vi "FPGA_Main_R3.vi"() -> ()   [LabVIEW 2018]
uses:
  Data Def/FPGA_I2C Loop State.ctl
  <vilib>/rvi/Emulation/niFpgaGetClockAttributes.vi
  <vilib>/rvi/Emulation/niFpgaSctlEmulationGetInTimedLoop.vi
  <vilib>/rvi/Emulation/niFpgaEmulationReportErrorSimple.vi
  <vilib>/IEDriver/SPIandI2C/FPGA/Private/Initialize Port (I2C).vi
  <vilib>/IEDriver/SPIandI2C/FPGA/Private/Configure Port (I2C).vi
  <vilib>/IEDriver/SPIandI2C/FPGA/Private/Read Port (I2C).vi
  <vilib>/IEDriver/SPIandI2C/FPGA/Private/Arm Port (I2C).vi
  <vilib>/IEDriver/SPIandI2C/FPGA/Private/Write Port (I2C).vi
  <vilib>/rvi/Emulation/niFpgaProcessEmulError.vi
  <vilib>/rvi/interface/RandomDataEmulation/niFpgaRandomDataHandleErrors.vi
  <vilib>/rvi/Emulation/niFpgaCriticalErrorInLSC.vi
  <vilib>/IEDriver/SPIandI2C/FPGA/Private/IP Port (I2C).vi
  <vilib>/rvi/DataTransferAndStorage/Container/XNode/niFpgaContainer.xnode
  <vilib>/rvi/interface/RandomDataEmulation/nirviRandomDataFpgaReadWriteTemplate.vi
  <vilib>/IEDriver/SPIandI2C/FPGA/Library/IP SPI&I2C.lvlib
panel:
  out "Count":u32
  out "I2C Loop State View":T1
  out "Over":bool
  in  "Auto Read Count":u32
  out "Overflow":bool
  in  "I2C Loop State":T1
  out "Done":bool
  in  "Command Data":T2 {"Command (Write & Read)" items=["Write & Read", "Write", "Read"]}
  out "Actual Rate (Hz)":u32
  in  "I2C Protocol Input Data":u8
  out "I2C Protocol Output Data":u8
  in  "I2C Protocol Configure":T3
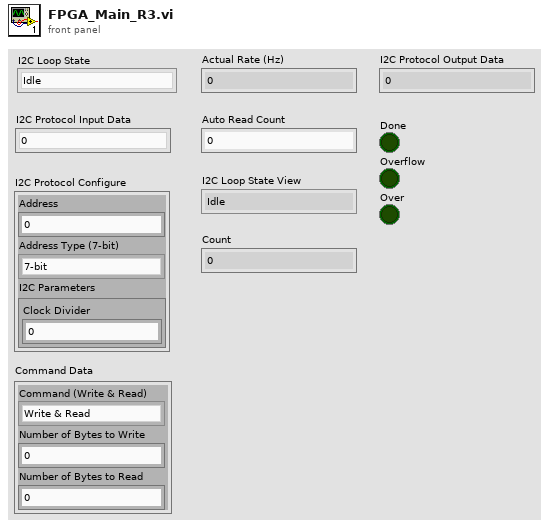
[diagram p1: front panel]
types:
  T1 = typedef "FPGA_I2C Loop State.ctl" = enum16{"Idle", "Set Idle", "Config", "Read", "Write", "Arm", "Auto Run", "Auto Config", "Auto Write", "Auto Arm", "Auto Read", "Auto Check"}
  T2 = cluster{"Command (Write & Read)":u8, "Number of Bytes to Write":u16, "Number of Bytes to Read":u16}
  T3 = cluster{"Address":u16, "Address Type (7-bit)":enum16{"7-bit", "10-bit"}, "I2C Parameters":cluster{"Clock Divider":u32}}
  T4 = typedef "IP SPI&I2C.lvlib/Private Data (I2C).ctl" = cluster{"Arm Trigger":refnum<k21>, "API to IP Data":refnum<k21>, "IP to API Data":refnum<k21>, "Configuration Register":refnum<k21>, "Configuration Lock":refnum<k21>}
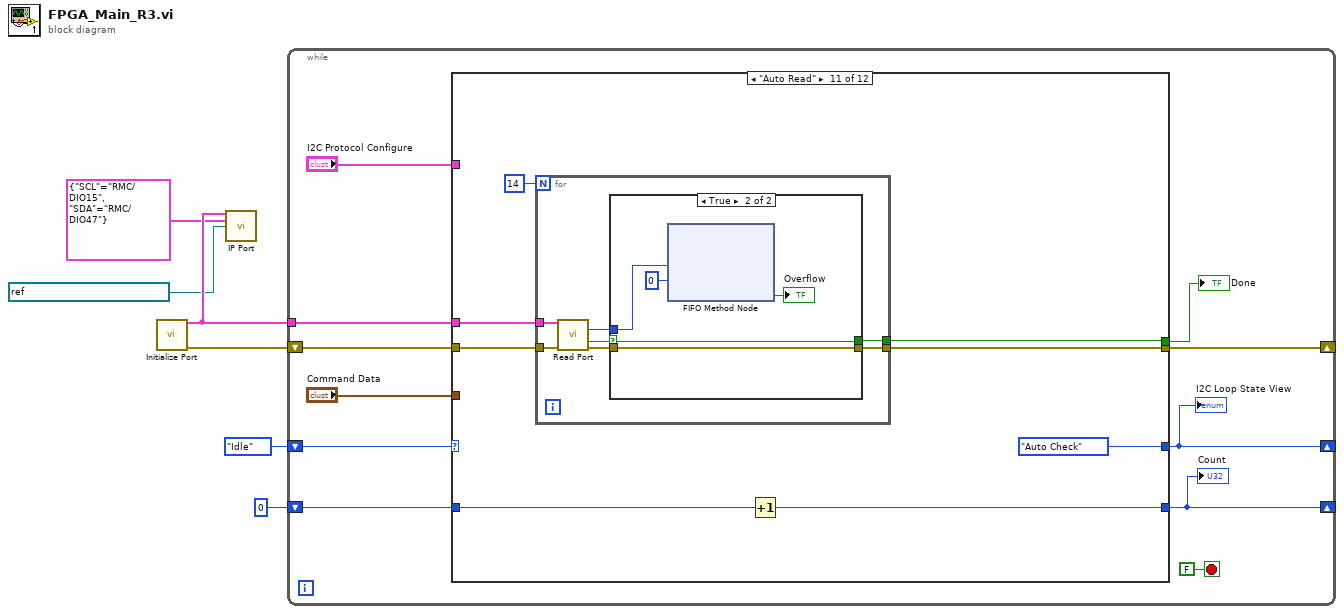
[diagram p0: block diagram]
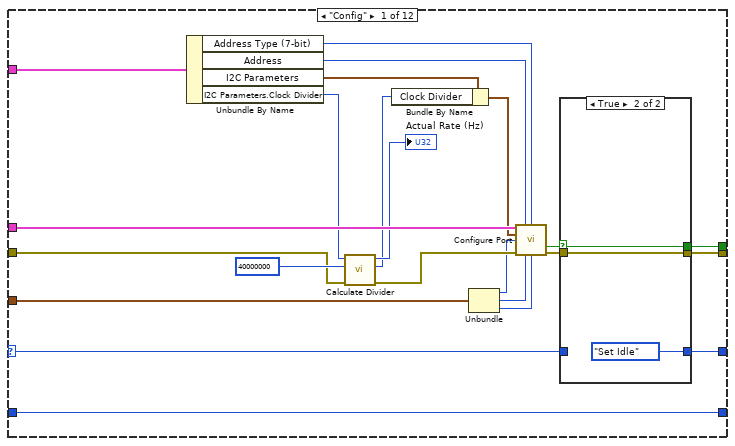
[diagram p2: hidden frame]
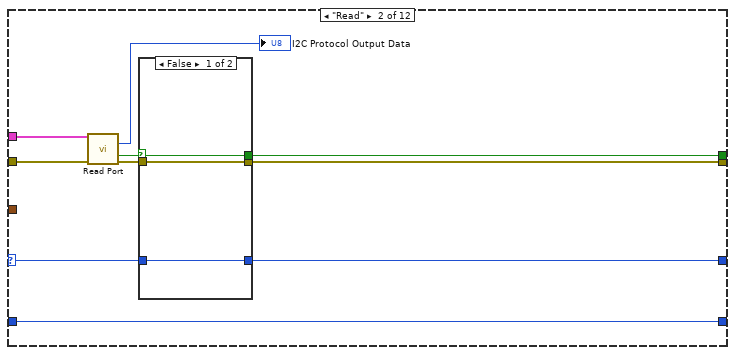
[diagram p4: hidden frame]
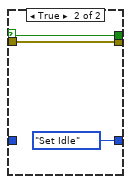
[diagram p5: hidden frame]
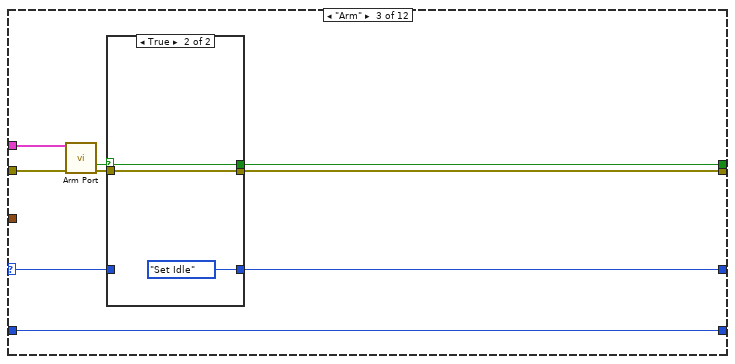
[diagram p6: hidden frame]
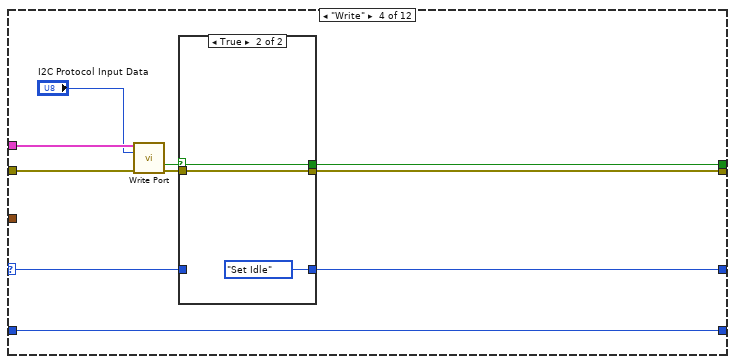
[diagram p8: hidden frame]
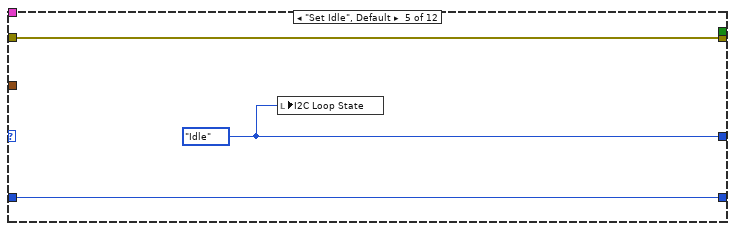
[diagram p10: hidden frame]
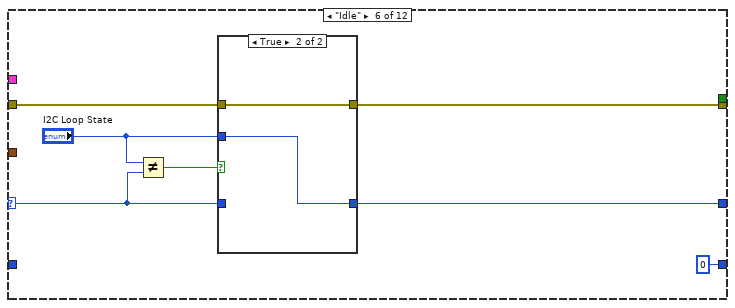
[diagram p11: hidden frame]
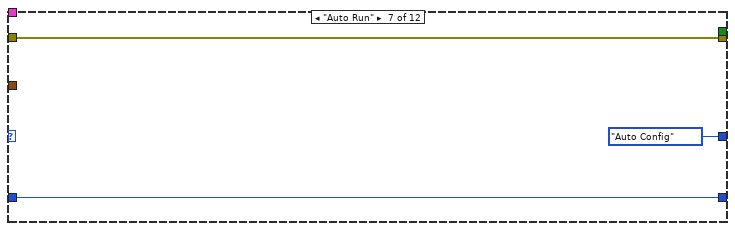
[diagram p13: hidden frame]
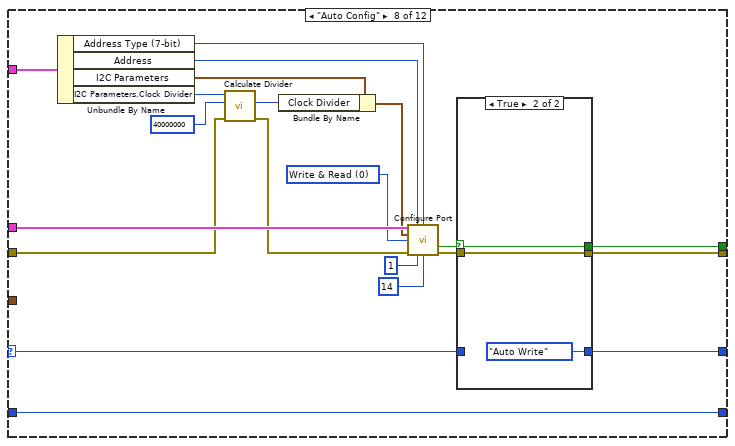
[diagram p14: hidden frame]
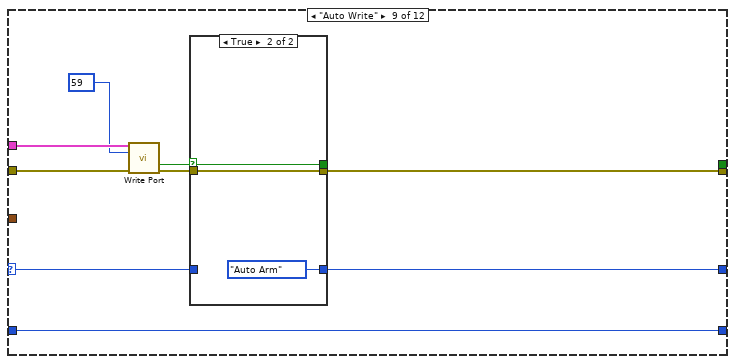
[diagram p16: hidden frame]
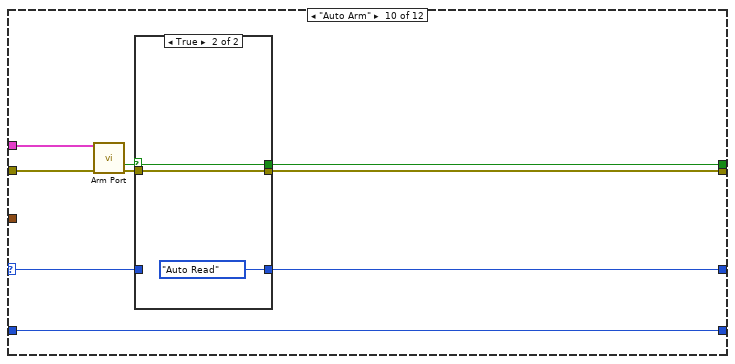
[diagram p18: hidden frame]
diagram:
  n1 = call-poly <vilib>:"Initialize Port.vi"() -> ("Private Data Out"=w5:T4, "error out"=w6:errorcluster)  [unwired: 14 in]
  n2 = call-poly <vilib>:"IP Port.vi"("Private Data In"=w5, "I2C FPGA IO"=cluster{"SCL":refnum<k21>, "SDA":refnum<k21>} {"SCL"="RMC/DIO15", "SDA"="RMC/DIO47"}, "FPGA Clock"=refnum<k21> "40 MHz Onboard Clock") -> ()  [unwired: 13 in]
  n3 = while {
    shift-right: [w12] -> _
    shift-left: w6 -> [w16]
    tunnel: w5 -> [w17]
    shift-right: [w13] -> _
    shift-left: FPGA_I2C_Loop_State."Idle" ("I2C Loop State") -> [w14]
    shift-right: [w7] -> _
    shift-left: u32 0 -> [w8]
    stop <- FALSE stop-if-true
    n4 = case shown="\"Auto Read\"" w14 {
      selector: w14 -> [w32 w52 w67 w82 _ w100 _ w112 w141 w157 _ w198]
      tunnel: w17 -> [w40 w56 w71 w87 _ _ _ w131 w145 w158 w175 _]
      tunnel: w16 -> [w38 w55 w70 w86 w96 w102 w108 w128 w146 w159 w170 w196]
      tunnel: [w33 w49 w65 w80 w96 w101 w108 w115 w140 w156 w169 w195] -> w12
      tunnel: [w31 w50 w66 w81 w94 w99 FPGA_I2C_Loop_State."Auto Config" ("I2C Loop State") w113 w139 w154 FPGA_I2C_Loop_State."Auto Check" ("I2C Loop State") w194] -> w13
      tunnel: "Command Data" -> [w30 _ _ _ _ _ _ _ _ _ _ _]
      tunnel: [w20 w48 w64 w79 _ _ _ w114 _ w155 w168 _] -> w10
      tunnel: "I2C Protocol Configure" -> [w19 _ _ _ _ _ _ w129 _ _ _ _]
      tunnel: w8 -> [w18 w47 w63 w78 w95 _ w110 w111 w138 w153 w173 w193]
      tunnel: [w18 w47 w63 w78 w95 u32 0 w110 w111 w138 w153 w172 w197] -> w7
      frame "Config" {
        n5 = Unbundle By Name(w19) -> ("Address Type (7-bit)"=w29:enum16{"7-bit", "10-bit"}, "Address"=w28:u16, "I2C Parameters"=w26:cluster{"Clock Divider":u32}, "I2C Parameters.Clock Divider"=w27:u32)
        n6 = call <vilib>:"Calculate Divider.vi"("error in"=w38, "FPGA Clock (Hz)"=u32 40000000, "Clock Rate (Hz)"=w27) -> ("error out"=w36:errorcluster, "Clock Divider"=w25:u32, "Actual Rate (Hz)"=→"Actual Rate (Hz)":u32)  [unwired: 6 in]
        n7 = Bundle By Name(cluster=w26, "Clock Divider"=w25) -> (w24:cluster{"Clock Divider":u32})
        n8 = Unbundle(w30) -> ("Command (Write & Read)"=w23:u8, "Number of Bytes to Write"=w22:u16, "Number of Bytes to Read"=w21:u16)
        n9 = call-poly <vilib>:"Configure Port.vi"("Private Data In"=w40, "Address"=w28, "Address Type (7-bit)"=w29, "I2C Parameters"=w24, "Command (Write & Read)"=w23, "error in"=w36, "Number of Bytes to Write"=w22, "Number of Bytes to Read"=w21) -> ("Done"=w35:bool, "error out"=w34:errorcluster)  [unwired: 5 in, 1 out]
        n10 = case shown="True" w35 {
          selector: w35 -> [w41 w45]
          tunnel: w34 -> [w43 w46]
          tunnel: [w43 w46] -> w33
          tunnel: w32 -> [w42 _]
          tunnel: [w42 FPGA_I2C_Loop_State."Set Idle" ("I2C Loop State")] -> w31
          tunnel: [w41 w45] -> w20
          frame False {
          }
          frame True {
          }
        }
      }
      frame "Read" {
        n11 = call-poly <vilib>:"Read Port.vi"("Private Data In"=w56, "error in"=w55) -> ("Data Out"=→"I2C Protocol Output Data":u8, "Output Valid"=w53:bool, "error out"=w51:errorcluster)  [unwired: 10 in, 1 out]
        n12 = case shown="False" w53 {
          selector: w53 -> [w57 w61]
          tunnel: w52 -> [w59 _]
          tunnel: w51 -> [w58 w62]
          tunnel: [w59 FPGA_I2C_Loop_State."Set Idle" ("I2C Loop State")] -> w50
          tunnel: [w58 w62] -> w49
          tunnel: [w57 w61] -> w48
          frame False {
          }
          frame True {
          }
        }
      }
      frame "Arm" {
        n13 = call-poly <vilib>:"Arm Port.vi"("Private Data In"=w71, "error in"=w70) -> ("Done"=w69:bool, "error out"=w68:errorcluster)  [unwired: 11 in, 1 out]
        n14 = case shown="True" w69 {
          selector: w69 -> [w72 w76]
          tunnel: w68 -> [w73 w77]
          tunnel: w67 -> [w74 _]
          tunnel: [w74 FPGA_I2C_Loop_State."Set Idle" ("I2C Loop State")] -> w66
          tunnel: [w73 w77] -> w65
          tunnel: [w72 w76] -> w64
          frame False {
          }
          frame True {
          }
        }
      }
      frame "Write" {
        n15 = call-poly <vilib>:"Write Port.vi"("Private Data In"=w87, "Data In"="I2C Protocol Input Data", "error in"=w86) -> ("Done"=w83:bool, "error out"=w84:errorcluster)  [unwired: 10 in, 1 out]
        n16 = case shown="True" w83 {
          selector: w83 -> [w88 w92]
          tunnel: w84 -> [w89 w93]
          tunnel: w82 -> [w90 _]
          tunnel: [w90 FPGA_I2C_Loop_State."Set Idle" ("I2C Loop State")] -> w81
          tunnel: [w89 w93] -> w80
          tunnel: [w88 w92] -> w79
          frame False {
          }
          frame True {
          }
        }
      }
      frame "Set Idle", Default {
        w94 = FPGA_I2C_Loop_State."Idle" ("I2C Loop State")
        n17 = local write "I2C Loop State"(w94) -> ()
      }
      frame "Idle" {
        n18 = Not Equal?(x="I2C Loop State", y=w100) -> (x != y?=w103:bool)
        n19 = case shown="True" w103 {
          tunnel: w102 -> [w105 w107]
          tunnel: [w105 w107] -> w101
          tunnel: w100 -> [w104 _]
          tunnel: "I2C Loop State" -> [_ w106]
          tunnel: [w104 w106] -> w99
          frame False {
          }
          frame True {
          }
        }
      }
      frame "Auto Run" {
      }
      frame "Auto Config" {
        w120 = u8 0 items=["Write & Read", "Write", "Read"] ("Command (Write & Read)")
        n20 = Unbundle By Name(w129) -> ("Address Type (7-bit)"=w123:enum16{"7-bit", "10-bit"}, "Address"=w122:u16, "I2C Parameters"=w130:cluster{"Clock Divider":u32}, "I2C Parameters.Clock Divider"=w127:u32)
        n21 = call <vilib>:"Calculate Divider.vi"("error in"=w128, "FPGA Clock (Hz)"=u32 40000000, "Clock Rate (Hz)"=w127) -> ("error out"=w125:errorcluster, "Clock Divider"=w126:u32)  [unwired: 6 in, 1 out]
        n22 = Bundle By Name(cluster=w130, "Clock Divider"=w126) -> (w121:cluster{"Clock Divider":u32})
        n23 = call-poly <vilib>:"Configure Port.vi"("Private Data In"=w131, "Address"=w122, "Address Type (7-bit)"=w123, "I2C Parameters"=w121, "Command (Write & Read)"=w120, "error in"=w125, "Number of Bytes to Write"=u16 1, "Number of Bytes to Read"=u16 14) -> ("Done"=w116:bool, "error out"=w117:errorcluster)  [unwired: 5 in, 1 out]
        n24 = case shown="True" w116 {
          selector: w116 -> [w132 w136]
          tunnel: w117 -> [w134 w137]
          tunnel: [w134 w137] -> w115
          tunnel: w112 -> [w133 _]
          tunnel: [w133 FPGA_I2C_Loop_State."Auto Write" ("I2C Loop State")] -> w113
          tunnel: [w132 w136] -> w114
          frame False {
          }
          frame True {
          }
        }
      }
      frame "Auto Write" {
        n25 = call-poly <vilib>:"Write Port.vi"("Private Data In"=w145, "Data In"=u8 59, "error in"=w146) -> ("Done"=w143:bool, "error out"=w144:errorcluster)  [unwired: 10 in, 1 out]
        n26 = case shown="True" w143 {
          selector: w143 -> [w147 w151]
          tunnel: w144 -> [w148 w152]
          tunnel: w141 -> [w149 _]
          tunnel: [w149 FPGA_I2C_Loop_State."Auto Arm" ("I2C Loop State")] -> w139
          tunnel: [w148 w152] -> w140
          tunnel: [w147 w151] -> _
          frame False {
          }
          frame True {
          }
        }
      }
      frame "Auto Arm" {
        n27 = call-poly <vilib>:"Arm Port.vi"("Private Data In"=w158, "error in"=w159) -> ("Done"=w161:bool, "error out"=w160:errorcluster)  [unwired: 11 in, 1 out]
        n28 = case shown="True" w161 {
          selector: w161 -> [w162 w166]
          tunnel: w160 -> [w163 w167]
          tunnel: w157 -> [w164 _]
          tunnel: [w164 FPGA_I2C_Loop_State."Auto Read" ("I2C Loop State")] -> w154
          tunnel: [w163 w167] -> w156
          tunnel: [w162 w166] -> w155
          frame False {
          }
          frame True {
          }
        }
      }
      frame "Auto Read" {
        n29 = for {
          N: 14 -> [_]
          tunnel: w175 -> [w182]
          tunnel: w170 -> [w179]
          tunnel: [w177] -> w169
          tunnel: [w176] -> w168
          n30 = call-poly <vilib>:"Read Port.vi"("Private Data In"=w182, "error in"=w179) -> ("Data Out"=w181:u8, "Output Valid"=w180:bool, "error out"=w178:errorcluster)  [unwired: 10 in, 1 out]
          n31 = case shown="True" w180 {
            selector: w180 -> [w184 w185]
            tunnel: w181 -> [_ w189]
            tunnel: w178 -> [w183 w186]
            tunnel: [w183 w186] -> w177
            tunnel: [w184 w185] -> w176
            frame False {
            }
            frame True {
              n32 = xnode ("FIFO Method Node")("Element"=w189, "Timeout"=0) -> ("Timed Out?"=→"Overflow":bool)  [unwired: 1 in, 1 out]
            }
          }
        }
        n33 = Increment(x=w173) -> (x+1=w172:u32)
      }
      frame "Auto Check" {
        n34 = Greater Or Equal?(x=w193, y="Auto Read Count") -> (x >= y?=w191:bool)
        n35 = case shown="False" w191 {
          selector: w191 -> [w199 w203]
          tunnel: w198 -> [_ _]
          tunnel: w193 -> [w202 w206]
          tunnel: [w202 w206] -> w197
          tunnel: w196 -> [w201 w205]
          tunnel: [w201 w205] -> w195
          tunnel: [FPGA_I2C_Loop_State."Auto Run" ("I2C Loop State") FPGA_I2C_Loop_State."Set Idle" ("I2C Loop State")] -> w194
          tunnel: [w199 w203] -> w190
          frame False {
          }
          frame True {
          }
        }
        "Over" <- w190
      }
    }
    "Done" <- w10
    "I2C Loop State View" <- w13
    "Count" <- w7
  }
